vi "externalSetParam.vi"(0 "reference":refnum<class "ClassRelationshipEdge.lvclass">, 1 "arrowHead":T1, 2 "string":string, 3 "node":refnum<class "AbstractNode.lvclass">, 4 "bentStyle":T2, 5 "error in (no error)":errorcluster, 6 "setParam":T3) -> (14 "reference out":refnum<class "ClassRelationshipEdge.lvclass">, 19 "error out":errorcluster)   [LabVIEW 2014, in "ClassRelationshipEdge.lvclass"]
doc: "Sets externaly parameters on object"
uses:
  <resource>/Framework/Providers/Open_GDS/UML/ClassRelationshipEdge_class/ClassRelationshipEdge.lvclass
  <resource>/Framework/Providers/Open_GDS/UML/ClassRelationshipEdge_class/ExternaSetParamType.ctl
  <resource>/Framework/Providers/Open_GDS/UML/AbstractNode_class/AbstractNode.lvclass
  <resource>/Framework/Providers/Open_GDS/UML/BentStyle_class/BentStyleType.ctl
  <resource>/Framework/Providers/Open_GDS/UML/ArrowHead_class/ArrowHeadType.ctl
  <resource>/Framework/Providers/Open_GDS/UML/ArrowHead_class/ArrowHead.lvclass
  <resource>/Framework/Providers/Open_GDS/UML/BentStyle_class/BentStyle.lvclass
  <resource>/Framework/Providers/Open_GDS/UML/SegmentedLineEdge_class/SegmentedLineEdge.lvclass
  <resource>/Framework/Providers/Open_GDS/UML/AbstractEdge_class/AbstractEdge.lvclass
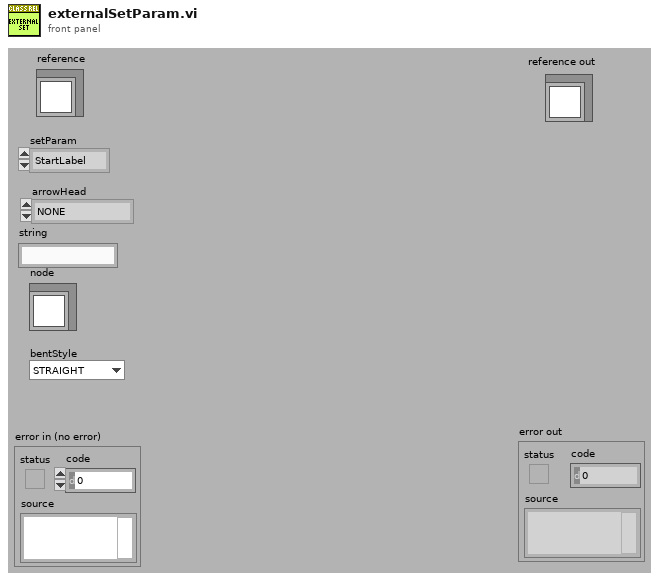
[diagram p1: front panel]
types:
  T1 = typedef "ArrowHead.lvclass/ArrowHeadType.ctl" = enum16{"NONE", "TRIANGLE", "BLACK_TRIANGLE", "V", "HALF_V", "DIAMOND", "BLACK_DIAMOND"}
  T2 = typedef "BentStyle.lvclass/BentStyleType.ctl" = enum16{"STRAIGHT", "HV", "VH", "HVH", "VHV", "ARC"}
  T3 = typedef "ClassRelationshipEdge.lvclass/ExternaSetParamType.ctl" = enum16{"StartLabel", "MidLabel", "EndLabel", "StartNode", "EndNode", "BendType", "StartArrow", "EndArrow"}
  T4 = typedef "ClassRelationshipEdge.lvclass/ObjectAttributes.ctl" = cluster{"bentStyleRef":refnum<class "BentStyle.lvclass">, "startConnectionOffset":cluster{"x":i32, "y":i32}, "endConnectionOffset":cluster{"x":i32, "y":i32}, "MidLineOffset":cluster{"x":i32, "y":i32}, "DepClass":T5}
  T5 = typedef "ReversedEngineering_ViDependencyDetailsType.ctl" = cluster{"ThisVIs/Ctls":path[], "Dependent_VIs/Ctls":path[]}
  T6 = typedef "SegmentedLineEdge.lvclass/ObjectAttributes.ctl" = cluster{"lineStyle":refnum<class "LineStyle.lvclass">, "startArrowHead":refnum<class "ArrowHead.lvclass">, "endArrowHead":refnum<class "ArrowHead.lvclass">, "startLabel":string, "midLabel":string, "endLabel":string, "MidLabelOffset":T7, "SplitWire":bool}
  T7 = typedef "Point Point2D.ctl" = cluster{"x":dbl, "y":dbl}
  T8 = typedef "AbstractEdge.lvclass/ObjectAttributes.ctl" = cluster{"start":refnum<class "AbstractNode.lvclass">, "end":refnum<class "AbstractNode.lvclass">}
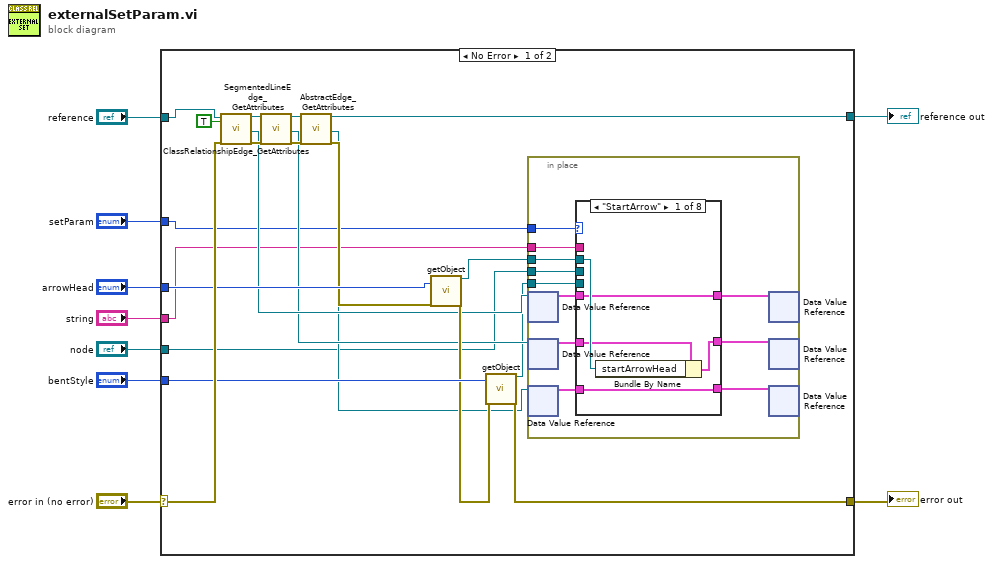
[diagram p0: block diagram]
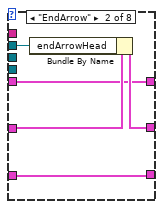
[diagram p2: hidden frame]
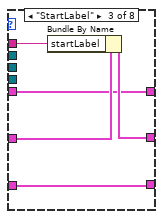
[diagram p3: hidden frame]
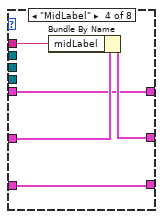
[diagram p4: hidden frame]
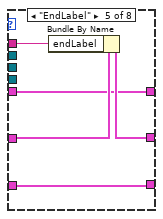
[diagram p5: hidden frame]
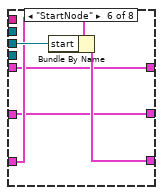
[diagram p6: hidden frame]
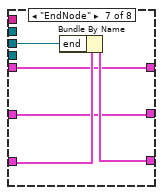
[diagram p7: hidden frame]
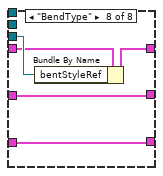
[diagram p8: hidden frame]
diagram:
  n1 = case shown="No Error" "error in (no error)" {
    selector: "error in (no error)" -> [w30 w82]
    tunnel: "reference" -> [w29 w83]
    tunnel: [w28 w82] -> w7
    tunnel: [w27 w83] -> w6
    tunnel: "setParam" -> [w14 _]
    tunnel: "string" -> [w13 _]
    tunnel: "arrowHead" -> [w26 _]
    tunnel: "node" -> [w11 _]
    tunnel: "bentStyle" -> [w25 _]
    frame No Error {
      n2 = call <resource>:"ClassRelationshipEdge_GetAttributes.vi"("reference in"=w29, "OnlyGetDvrReference(False)"=TRUE, "error in (no error)"=w30) -> ("reference out"=w22:refnum<class "ClassRelationshipEdge.lvclass">, "DataRef"=w17:refnum<data-value>, "error out"=w21:errorcluster)  [unwired: 13 in, 1 out]
      n3 = call <resource>:"SegmentedLineEdge_GetAttributes.vi"("reference in"=w22, "error in (no error)"=w21) -> ("reference out"=w20:refnum<class "ClassRelationshipEdge.lvclass">, "DataRef"=w16:refnum<data-value>, "error out"=w19:errorcluster)  [unwired: 14 in, 1 out]
      n4 = call <resource>:"AbstractEdge_GetAttributes.vi"("reference in"=w20, "error in (no error)"=w19) -> ("reference out"=w27:refnum<class "ClassRelationshipEdge.lvclass">, "DataRef"=w15:refnum<data-value>, "error out"=w18:errorcluster)  [unwired: 14 in, 1 out]
      n5 = call <resource>:"getObject.vi"("arrowHead"=w26, "error in (no error)"=w18) -> ("reference out"=w12:refnum<class "ArrowHead.lvclass">, "error out"=w24:errorcluster)  [unwired: 16 out]
      n6 = call <resource>:"getObject.vi"("bentStyle"=w25, "error in (no error)"=w24) -> ("reference out"=w10:refnum<class "BentStyle.lvclass">, "error out"=w28:errorcluster)  [unwired: 16 out]
      n7 = in-place {
        in-place-border: w14 -> [w41]
        in-place-border: w13 -> [w40]
        in-place-border: w12 -> [w39]
        in-place-border: w11 -> [w38]
        in-place-border: w10 -> [w37]
        n8 = in-place-dvr #1(w17) -> (w34:T4)  [unwired: 1 out]
        n9 = in-place-dvr #2(w16) -> (w36:T6)  [unwired: 1 out]
        n10 = in-place-dvr #3(w15) -> (w35:T8)  [unwired: 1 out]
        n11 = case shown="\"StartArrow\"" w41 {
          tunnel: [w46 w49 w56 w61 w66 w68 w72 w77] -> w33
          tunnel: w40 -> [_ _ w55 w60 w65 _ _ _]
          tunnel: w39 -> [w45 w51 _ _ _ _ _ _]
          tunnel: w38 -> [_ _ _ _ _ w71 w76 _]
          tunnel: w37 -> [_ _ _ _ _ _ _ w81]
          tunnel: w36 -> [w44 w50 w54 w59 w64 w68 w72 w77]
          tunnel: w35 -> [w43 w48 w53 w58 w63 w70 w75 w78]
          tunnel: w34 -> [w42 w47 w52 w57 w62 w67 w73 w80]
          tunnel: [w43 w48 w53 w58 w63 w69 w74 w78] -> w32
          tunnel: [w42 w47 w52 w57 w62 w67 w73 w79] -> w31
          frame "StartArrow" {
            n12 = Bundle By Name(cluster=w44, "startArrowHead"=w45) -> (w46:T6)
          }
          frame "EndArrow" {
            n13 = Bundle By Name(cluster=w50, "endArrowHead"=w51) -> (w49:T6)
          }
          frame "StartLabel" {
            n14 = Bundle By Name(cluster=w54, "startLabel"=w55) -> (w56:T6)
          }
          frame "MidLabel" {
            n15 = Bundle By Name(cluster=w59, "midLabel"=w60) -> (w61:T6)
          }
          frame "EndLabel" {
            n16 = Bundle By Name(cluster=w64, "endLabel"=w65) -> (w66:T6)
          }
          frame "StartNode" {
            n17 = Bundle By Name(cluster=w70, "start"=w71) -> (w69:T8)
          }
          frame "EndNode" {
            n18 = Bundle By Name(cluster=w75, "end"=w76) -> (w74:T8)
          }
          frame "BendType" {
            n19 = Bundle By Name(cluster=w80, "bentStyleRef"=w81) -> (w79:T4)
          }
        }
        n20 = in-place-dvr #1(w31) -> ()  [unwired: 2 out]
        n21 = in-place-dvr #2(w33) -> ()  [unwired: 2 out]
        n22 = in-place-dvr #3(w32) -> ()  [unwired: 2 out]
      }
    }
    frame Error {
    }
  }
  "reference out" <- w6
  "error out" <- w7
